vi "后台任务.vi"(11 "Event In":refnum<class "NISAST Event.lvclass">) -> ()   [LabVIEW 2013]
uses:
  <resource>/importtools/Common/Event/NISAST Event.lvclass
  <vilib>/Platform/TimedLoop/XDataNode/timing_clust.ctl
  <vilib>/Platform/TimedLoop/XDataNode/nitl_modes.ctl
  <vilib>/Platform/TimedLoop/XDataNode/wakeup.ctl
  <vilib>/Platform/TimedLoop/XDataNode/XDataNode.xnode
  <vilib>/Platform/TimedLoop/XDataNode/XDNodeRunTimeDep.lvlib
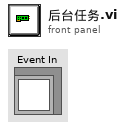
[diagram p1: front panel]
types:
  T1 = typedef "XDNodeRunTimeDep.lvlib/timing_clust.ctl" = cluster{"Expected End [f-1]":u64, "Actual End [f-1]":u64, "Finished Late? [f-1]":bool, "Expected End [i-1]":u64, "Actual End [i-1]":u64, "Finished Late? [i-1]":bool, "Expected Start [i]":u64, "Actual Start [i]":u64, "Expected Start [f]":u64, "Actual Start [f]":u64, "Source Name":string, "Structure Name":string, "Period":i64, "Deadline":i64, "Offset":i64, "Start":i64, "Priority":i32, "Timeout":i32, "Mode":T2, "Wakeup Reason":T3, "Error":errorcluster, "Source Type":string, "Secondary Source Type":string, "Global End Time":u64, "Global Start Time":u64, "Frame Duration":u64, "Iteration Duration":u64, "Assigned CPU":i32, "I/O Scan Engine Mode":u32}
  T2 = typedef "XDNodeRunTimeDep.lvlib/nitl_modes.ctl" = enum32{"No Change", "Process missed periods, maintain original phase", "Discard missed periods, maintain original phase", "Process missed periods, ignore original phase", "Discard missed periods, ignore original phase"}
  T3 = typedef "XDNodeRunTimeDep.lvlib/wakeup.ctl" = enum32{"Normal", "Aborted", "Asynchronous wakeup", "Timing source error", "Timed loop error", "Timeout"}
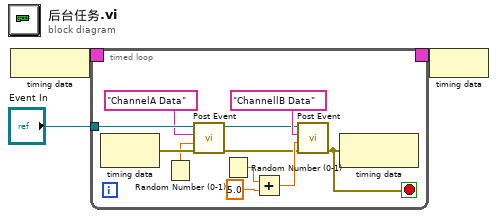
[diagram p0: block diagram]
diagram:
  n1 = node-c288() -> (w3:T1)
  n2 = timed-loop {
    timing: w3 -> [_]
    timing-out: [_] -> w2
    tunnel: "Event In" -> [w14]
    stop <- w4 stop-if-true
    n3 = node-c288() -> (w13:errorcluster)  [unwired: 1 in]
    n4 = Random Number (0-1)() -> (number: 0 to 1=w11:dbl)
    n5 = call-dynamic "Post Event.vi"("error in (no error)"=w13, "Event Data"=w11, "Event Name"="ChannelA Data", "Event in"=w14) -> ("error out"=w5:errorcluster, "Event out"=w6:refnum<class "NISAST Event.lvclass">)  [unwired: 6 in]
    n6 = Random Number (0-1)() -> (number: 0 to 1=w10:dbl)
    n7 = Add(x=w10, y=5.0) -> (x+y=w8:dbl)
    n8 = call-dynamic "Post Event.vi"("error in (no error)"=w5, "Event Data"=w8, "Event Name"="ChannellB Data", "Event in"=w6) -> ("error out"=w4:errorcluster)  [unwired: 6 in, 1 out]
    n9 = node-c288(w4) -> ()  [unwired: 1 out]
  }
  n10 = node-c288(w2) -> ()
